vi "Control_SR7265.vi"() -> ()   [LabVIEW 2015]
panel:
  in  "Record new values":bool
  out "Y (V)":dbl
  out "X (V)":dbl
  out "Harmonic #":i32
  out "Phase":dbl
  out "Oscillator (V)":dbl
  out "Frequency (Hz)":dbl
  out "Time Constant":u16(ring) items=["10 us", "20 us", "40 us", "80 us", "160 us", "320 us", "640 us", "5 ms", "10 ms", "20 ms", "50 ms", "100 ms", "200 ms", "500 ms", "1 s", "2 s", "5 s", "10 s", "20 s", "50 s", "100 s", "200 s", "500 s", "1 ks", "2 ks", "5 ks", "10 ks", "20 ks", "50 ks", "100 ks"]
  out "Sensitivity":u16(ring) items=["NA", "2 nV", "5 nV", "10 nV", "20 nV", "50 nV", "100 nV", "200 nV", "500 nV", "1 uV", "2 uV", "5 uV", "10 uV", "20 uV", "50 uV", "100 uV", "200 uV", "500 uV", "1 mV", "2 mV", "5 mV", "10 mV", "20 mV", "50 mV", "100 mV", "200 mV", "500 mV", "1 V"]
  in  "ON/OFF channel":bool
  in  "error in (no error)":errorcluster
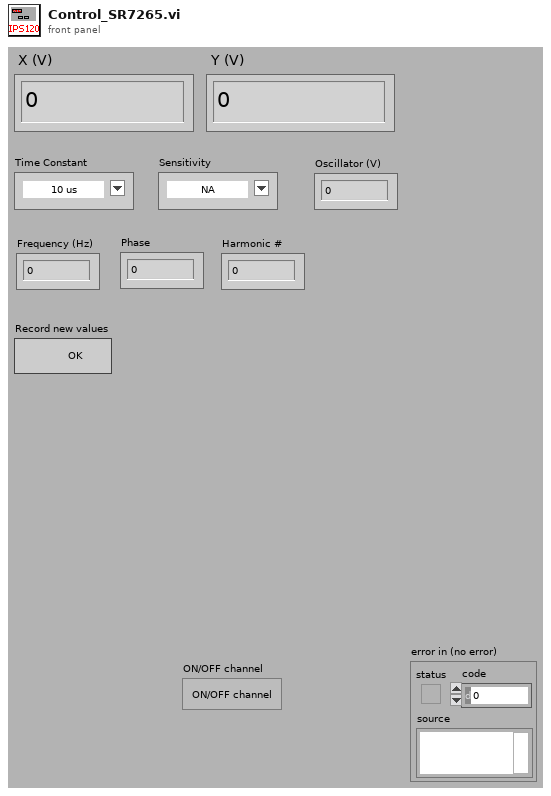
[diagram p1: front panel]
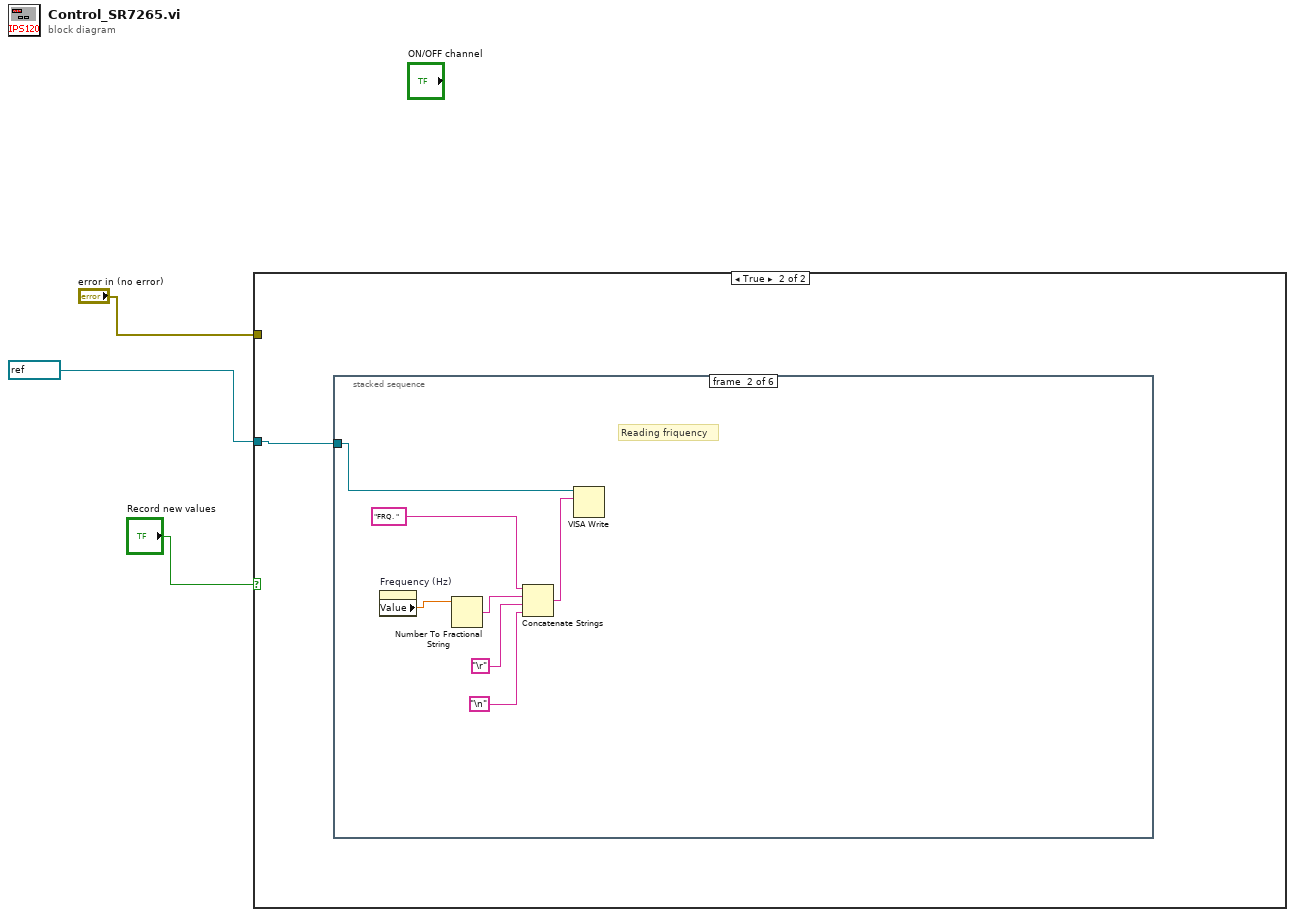
[diagram p0: block diagram]
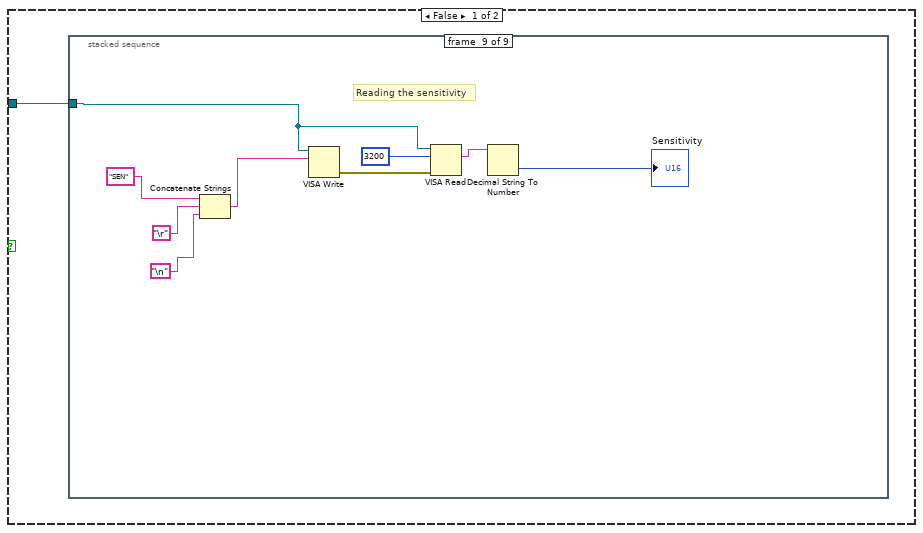
[diagram p2: hidden frame]
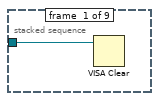
[diagram p3: hidden frame]
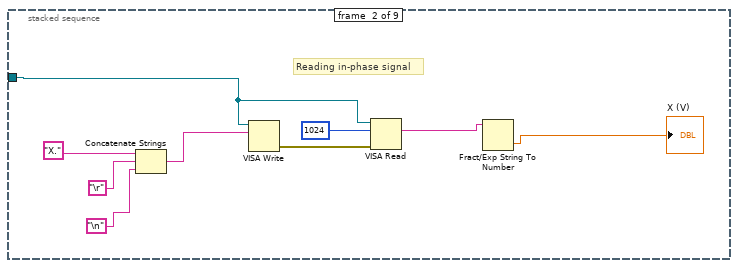
[diagram p4: hidden frame]
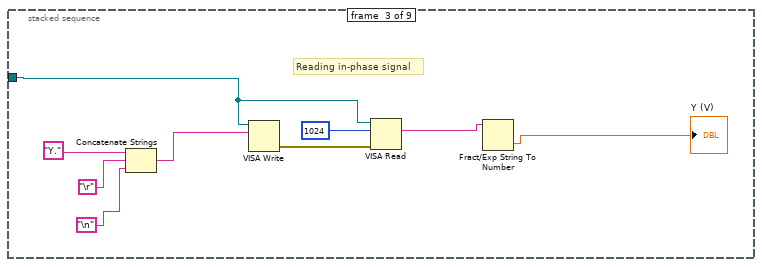
[diagram p5: hidden frame]
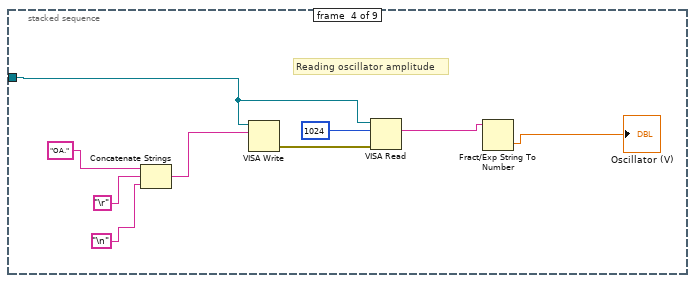
[diagram p6: hidden frame]
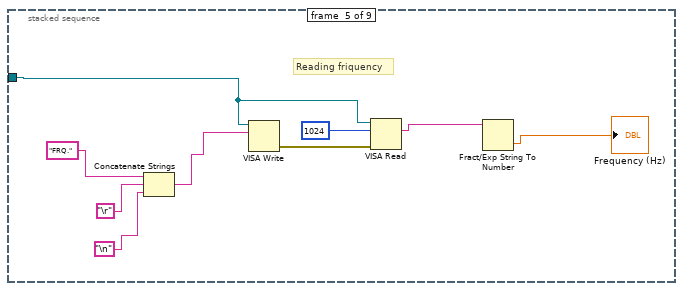
[diagram p7: hidden frame]
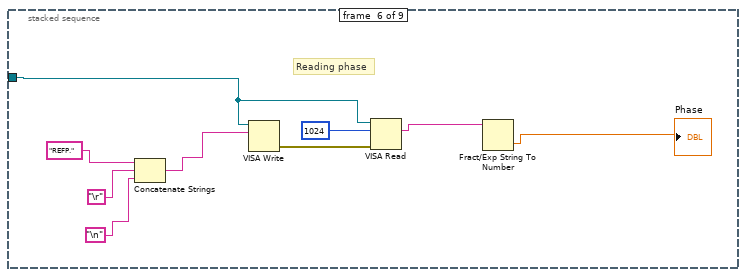
[diagram p8: hidden frame]
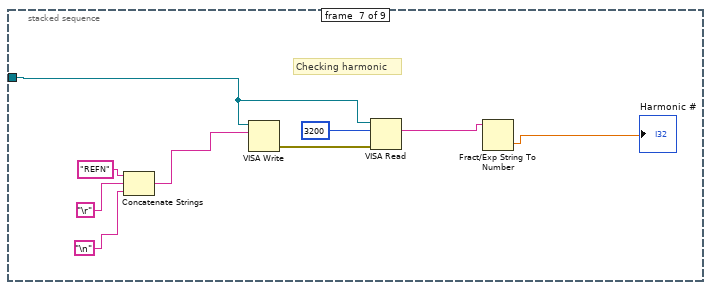
[diagram p9: hidden frame]
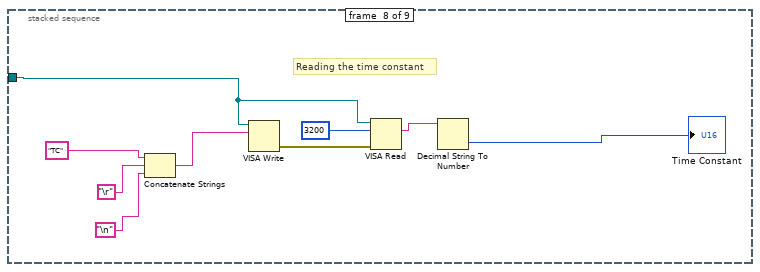
[diagram p10: hidden frame]
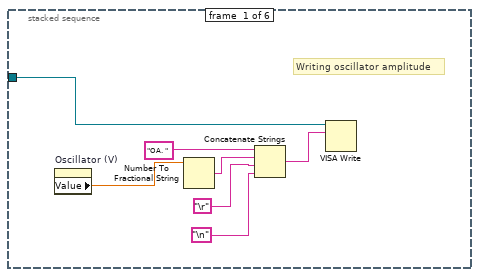
[diagram p11: hidden frame]
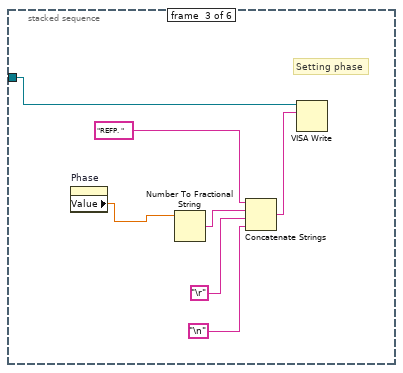
[diagram p12: hidden frame]
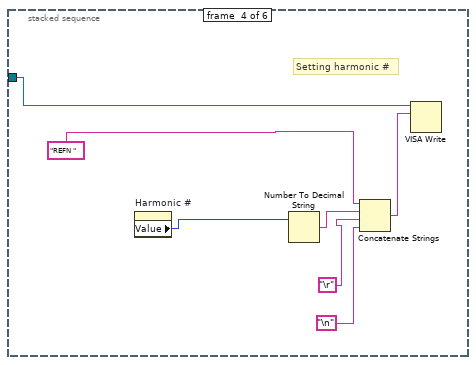
[diagram p13: hidden frame]
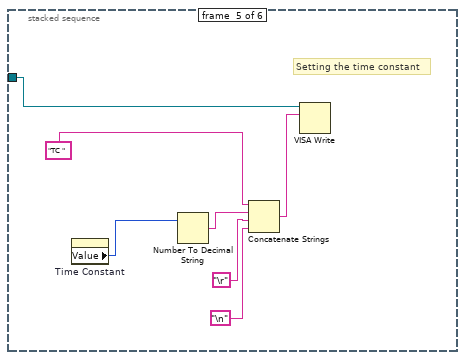
[diagram p14: hidden frame]
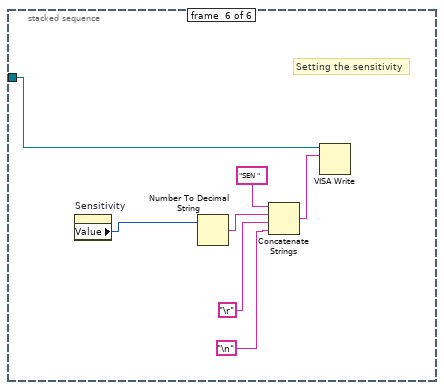
[diagram p15: hidden frame]
diagram:
  n1 = case shown="True" "Record new values" {
    tunnel: refnum<visa-resource-name> "7265" ("VISA resource name") -> [w4 w78]
    tunnel: "error in (no error)" -> [_ _]
    frame False {
      n2 = stacked-sequence {
        tunnel: w4 -> [w5 w11 w21 w29 w38 w47 w56 w65 w74]
        frame #0 {
          n3 = VISA Clear(VISA resource name=w5) -> ()  [unwired: 1 in, 2 out]
        }
        frame #1 {
          # "Reading in-phase signal"
          n4 = Concatenate Strings("X.", "\r", "\n") -> (w6:string)
          n5 = VISA Write(VISA resource name=w11, write buffer=w6) -> (error out=w14:errorcluster)  [unwired: 1 in, 2 out]
          n6 = VISA Read(VISA resource name=w11, byte count=u32 1024, error in (no error)=w14) -> (read buffer=w10:string)  [unwired: 3 out]
          n7 = Fract/Exp String To Number(string=w10) -> (number=→"X (V)":dbl)  [unwired: 3 in, 1 out]
        }
        frame #2 {
          # "Reading in-phase signal"
          n8 = Concatenate Strings("Y.", "\r", "\n") -> (w16:string)
          n9 = VISA Write(VISA resource name=w21, write buffer=w16) -> (error out=w23:errorcluster)  [unwired: 1 in, 2 out]
          n10 = VISA Read(VISA resource name=w21, byte count=u32 1024, error in (no error)=w23) -> (read buffer=w20:string)  [unwired: 3 out]
          n11 = Fract/Exp String To Number(string=w20) -> (number=→"Y (V)":dbl)  [unwired: 3 in, 1 out]
        }
        frame #3 {
          # "Reading oscillator amplitude"
          n12 = Concatenate Strings("OA.", "\r", "\n") -> (w24:string)
          n13 = VISA Write(VISA resource name=w29, write buffer=w24) -> (error out=w32:errorcluster)  [unwired: 1 in, 2 out]
          n14 = VISA Read(VISA resource name=w29, byte count=u32 1024, error in (no error)=w32) -> (read buffer=w28:string)  [unwired: 3 out]
          n15 = Fract/Exp String To Number(string=w28) -> (number=→"Oscillator (V)":dbl)  [unwired: 3 in, 1 out]
        }
        frame #4 {
          # "Reading friquency"
          n16 = Concatenate Strings("FRQ.", "\r", "\n") -> (w33:string)
          n17 = VISA Write(VISA resource name=w38, write buffer=w33) -> (error out=w41:errorcluster)  [unwired: 1 in, 2 out]
          n18 = VISA Read(VISA resource name=w38, byte count=u32 1024, error in (no error)=w41) -> (read buffer=w37:string)  [unwired: 3 out]
          n19 = Fract/Exp String To Number(string=w37) -> (number=→"Frequency (Hz)":dbl)  [unwired: 3 in, 1 out]
        }
        frame #5 {
          # "Reading phase"
          n20 = Concatenate Strings("REFP.", "\r", "\n") -> (w43:string)
          n21 = VISA Write(VISA resource name=w47, write buffer=w43) -> (error out=w50:errorcluster)  [unwired: 1 in, 2 out]
          n22 = VISA Read(VISA resource name=w47, byte count=u32 1024, error in (no error)=w50) -> (read buffer=w46:string)  [unwired: 3 out]
          n23 = Fract/Exp String To Number(string=w46) -> (number=→"Phase":dbl)  [unwired: 3 in, 1 out]
        }
        frame #6 {
          # "Checking harmonic"
          n24 = Concatenate Strings("REFN", "\r", "\n") -> (w52:string)
          n25 = VISA Write(VISA resource name=w56, write buffer=w52) -> (error out=w59:errorcluster)  [unwired: 1 in, 2 out]
          n26 = VISA Read(VISA resource name=w56, byte count=u32 3200, error in (no error)=w59) -> (read buffer=w51:string)  [unwired: 3 out]
          n27 = Fract/Exp String To Number(string=w51) -> (number=→"Harmonic #":dbl)  [unwired: 3 in, 1 out]
        }
        frame #7 {
          # "Reading the time constant"
          n28 = Concatenate Strings("TC", "\r", "\n") -> (w61:string)
          n29 = VISA Write(VISA resource name=w65, write buffer=w61) -> (error out=w68:errorcluster)  [unwired: 1 in, 2 out]
          n30 = VISA Read(VISA resource name=w65, byte count=u32 3200, error in (no error)=w68) -> (read buffer=w64:string)  [unwired: 3 out]
          n31 = Decimal String To Number(string=w64) -> (number=→"Time Constant":i32)  [unwired: 2 in, 1 out]
        }
        frame #8 {
          # "Reading the sensitivity"
          n32 = Concatenate Strings("SEN", "\r", "\n") -> (w70:string)
          n33 = VISA Write(VISA resource name=w74, write buffer=w70) -> (error out=w77:errorcluster)  [unwired: 1 in, 2 out]
          n34 = VISA Read(VISA resource name=w74, byte count=u32 3200, error in (no error)=w77) -> (read buffer=w73:string)  [unwired: 3 out]
          n35 = Decimal String To Number(string=w73) -> (number=→"Sensitivity":i32)  [unwired: 2 in, 1 out]
        }
      }
    }
    frame True {
      n36 = stacked-sequence {
        tunnel: w78 -> [w81 w88 w96 w102 w109 w116]
        frame #0 {
          # "Writing oscillator amplitude"
          n37 = property on="Oscillator (V)" class="DigNum (strict)"() -> ("Value"=w85:dbl)  [unwired: 2 in, 2 out]
          n38 = Number To Fractional String(number=w85) -> (F-format string=w84:string)  [unwired: 3 in]
          n39 = Concatenate Strings("OA. ", w84, "\r", "\n") -> (w83:string)
          n40 = VISA Write(VISA resource name=w81, write buffer=w83) -> ()  [unwired: 1 in, 3 out]
        }
        frame #1 {
          # "Reading friquency"
          n41 = property on="Frequency (Hz)" class="DigNum (strict)"() -> ("Value"=w90:dbl)  [unwired: 2 in, 2 out]
          n42 = Number To Fractional String(number=w90) -> (F-format string=w92:string)  [unwired: 3 in]
          n43 = Concatenate Strings("FRQ. ", w92, "\r", "\n") -> (w89:string)
          n44 = VISA Write(VISA resource name=w88, write buffer=w89) -> ()  [unwired: 1 in, 3 out]
        }
        frame #2 {
          # "Setting phase"
          n45 = property on="Phase" class="DigNum (strict)"() -> ("Value"=w95:dbl)  [unwired: 2 in, 2 out]
          n46 = Number To Fractional String(number=w95) -> (F-format string=w99:string)  [unwired: 3 in]
          n47 = Concatenate Strings("REFP. ", w99, "\r", "\n") -> (w97:string)
          n48 = VISA Write(VISA resource name=w96, write buffer=w97) -> ()  [unwired: 1 in, 3 out]
        }
        frame #3 {
          # "Setting harmonic #"
          n49 = property on="Harmonic #" class="DigNum (strict)"() -> ("Value"=w103:i32)  [unwired: 2 in, 2 out]
          n50 = Number To Decimal String(number=w103) -> (decimal integer string=w106:string)  [unwired: 1 in]
          n51 = Concatenate Strings("REFN ", w106, "\r", "\n") -> (w105:string)
          n52 = VISA Write(VISA resource name=w102, write buffer=w105) -> ()  [unwired: 1 in, 3 out]
        }
        frame #4 {
          # "Setting the time constant"
          n53 = property on="Time Constant" class="Ring (strict)"() -> ("Value"=w110:u16)  [unwired: 2 in, 2 out]
          n54 = Number To Decimal String(number=w110) -> (decimal integer string=w113:string)  [unwired: 1 in]
          n55 = Concatenate Strings("TC ", w113, "\r", "\n") -> (w112:string)
          n56 = VISA Write(VISA resource name=w109, write buffer=w112) -> ()  [unwired: 1 in, 3 out]
        }
        frame #5 {
          # "Setting the sensitivity"
          n57 = property on="Sensitivity" class="Ring (strict)"() -> ("Value"=w117:u16)  [unwired: 2 in, 2 out]
          n58 = Number To Decimal String(number=w117) -> (decimal integer string=w120:string)  [unwired: 1 in]
          n59 = Concatenate Strings("SEN ", w120, "\r", "\n") -> (w119:string)
          n60 = VISA Write(VISA resource name=w116, write buffer=w119) -> ()  [unwired: 1 in, 3 out]
        }
      }
    }
  }
